vi "Digital Write.vi"() -> ()   [LabVIEW 2009]
panel:
  in  "stop":bool
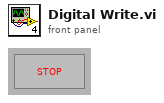
[diagram p1: front panel]
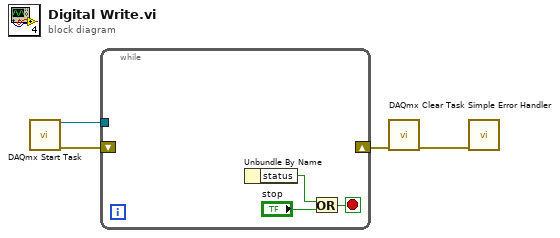
[diagram p0: block diagram]
diagram:
  n1 = call <vilib>:"DAQmx Start Task.vi"() -> ("task out"=w4:refnum<k21>, "error out"=w3:errorcluster)  [unwired: 14 in]
  n2 = while {
    tunnel: w4 -> [_]
    shift-right: [_] -> w2
    shift-left: w3 -> [_]
    stop <- w5 stop-if-true
    n3 = Unbundle By Name "Unbundle By Name"() -> ("status"=w7:bool)  [unwired: 1 in]
    n4 = Or(x=w7, y="stop") -> (x .or. y?=w5:bool)
  }
  n5 = call <vilib>:"DAQmx Clear Task.vi"("error in"=w2) -> ("error out"=w1:errorcluster)  [unwired: 14 in]
  n6 = call <vilib>:"Simple Error Handler.vi"("error in (no error)"=w1) -> ()  [unwired: 4 in, 5 out]
